vi "EventRegister_SetOPC.vi"(8 "Fehler (Eingang, kein Fehler)":errorcluster caption="Error_In", 11 "OXYGEN Ref In":refnum<visa-resource-name>) -> (0 "Fehler (Ausgang)":errorcluster caption="Error_Out", 1 "communication_data":T1, 3 "OXYGEN Ref Out":refnum<visa-resource-name>)   [LabVIEW 2018, in "OXYGEN.lvlib"]
doc: "Sets bit 0 (OPC bit) of the standard event register to 1 upon the completion of the specified overlap command."
uses:
  OXYGEN.lvlib
  TypeDefs/Cluster_RawCommData.ctl
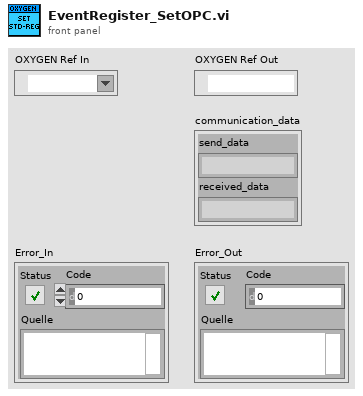
[diagram p1: front panel]
types:
  T1 = typedef "OXYGEN.lvlib/Cluster_RawCommData.ctl" = cluster{"send_data":string, "received_data":string}
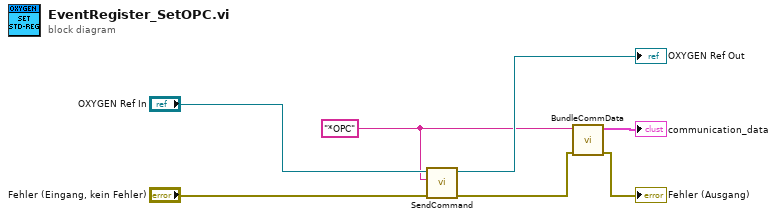
[diagram p0: block diagram]
diagram:
  w4 = "*OPC" ("Schreibpuffer")
  n1 = call "SendCommand.vi"("error in (no error)"="Fehler (Eingang, kein Fehler)", "String to Send"=w4, "OXY_SCPI Reseource In"="OXYGEN Ref In") -> ("error out"=w2:errorcluster, "OXY_SCPI Reseource Out"=→"OXYGEN Ref Out":refnum<visa-resource-name>)  [unwired: 7 in]
  n2 = call "BundleCommData.vi"("error in (no error)"=w2, "send_data"=w4) -> ("error out"=→"Fehler (Ausgang)":errorcluster, "communication_data"=→"communication_data":T1)  [unwired: 8 in]
